vi "Copy Image Section.vi"(8 "Error In":errorcluster, 9 "Index to Copy (row, column)":cluster{"x":i16, "y":i16}, 10 "Pasteboard Picture":picture, 11 "Copy Picture":picture) -> (0 "Error Out":errorcluster, 3 "Output Picture":picture)   [LabVIEW 2011]
doc: "Copies a 50px by 50px box specified by a (row, column) index over a copy of the pasteboard picture onto a new picture."
panel:
  # "50px x 50px Subset"
  # "+"
  # "="
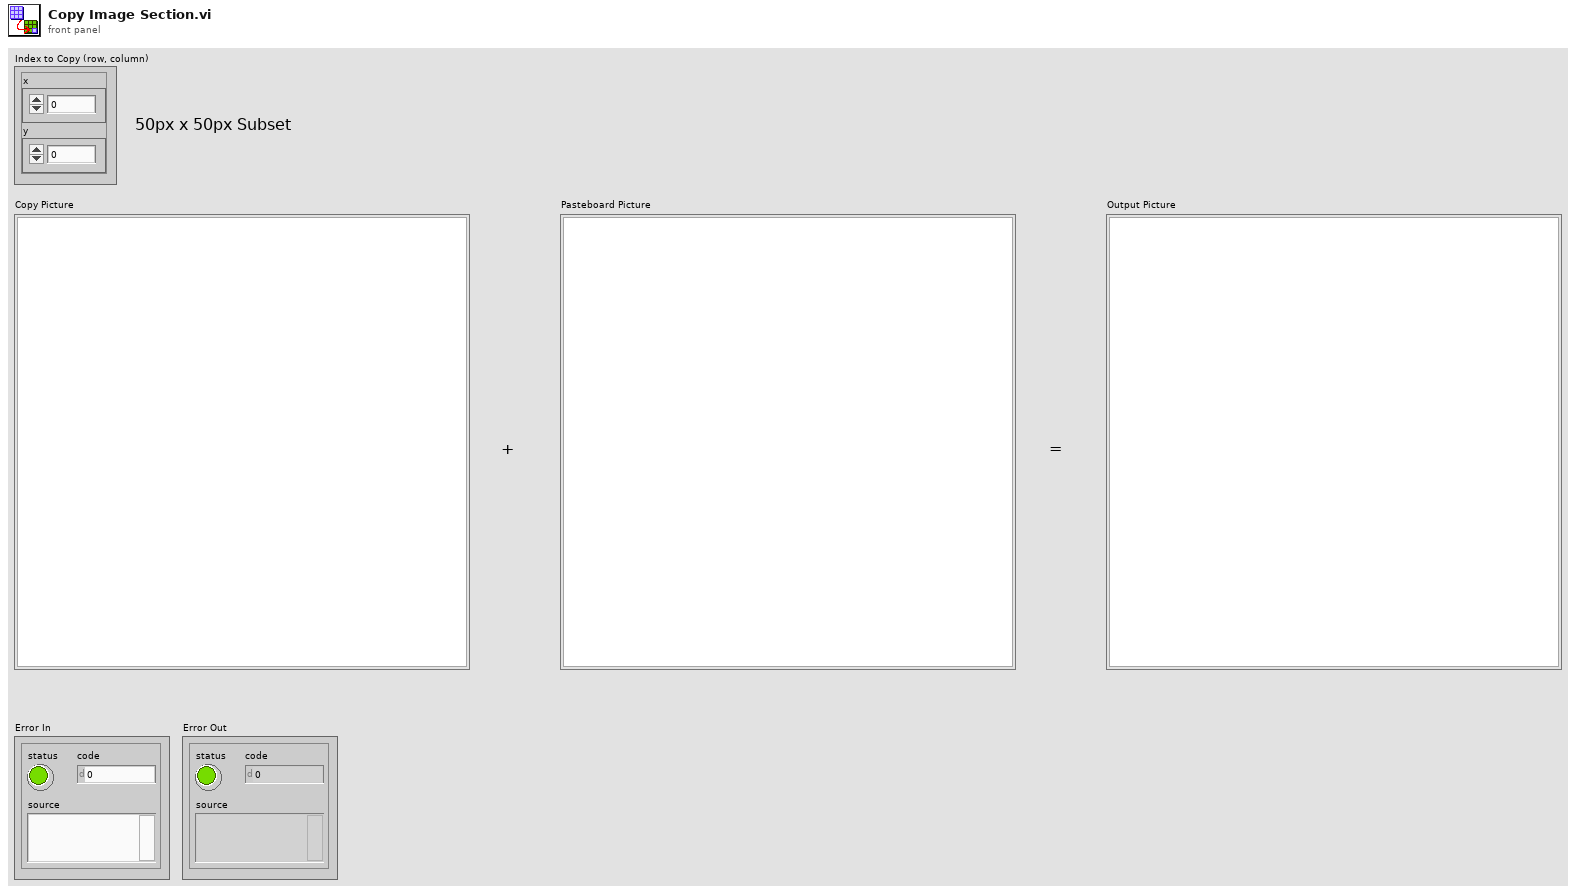
[diagram p1: front panel]
types:
  T1 = cluster{"left":i16, "top":i16, "right":i16, "bottom":i16}
  T2 = typedef "imagedata.ctl" = cluster{"image type":i32, "image depth":i32, "image":u8[], "mask":u8[], "colors":u32[], "Rectangle":cluster{"left":i16, "top":i16, "right":i16, "bottom":i16}}
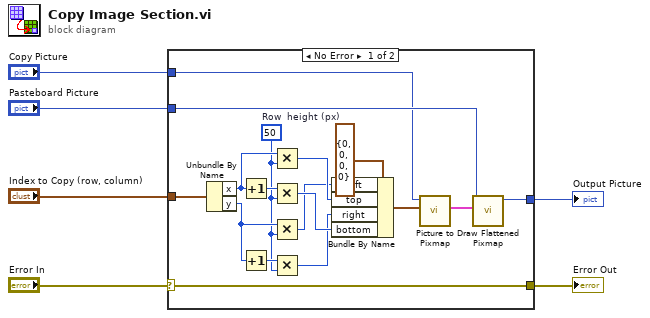
[diagram p0: block diagram]
diagram:
  n1 = case shown="No Error" "Error In" {
    selector: "Error In" -> [w7 w24]
    tunnel: "Index to Copy (row, column)" -> [w23 _]
    tunnel: "Pasteboard Picture" -> [w11 w25]
    tunnel: [w9 w25] -> w4
    tunnel: "Copy Picture" -> [w8 _]
    tunnel: [w7 w24] -> w1
    frame No Error {
      w18 = i16 50  # Row  height (px)
      n2 = Unbundle By Name(w23) -> ("x"=w22:i16, "y"=w20:i16)
      n3 = Increment(x=w22) -> (x+1=w21:i16)
      n4 = Increment(x=w20) -> (x+1=w19:i16)
      n5 = Multiply(x=w22, y=w18) -> (x*y=w17:i16)
      n6 = Multiply(x=w21, y=w18) -> (x*y=w16:i16)
      n7 = Multiply(x=w20, y=w18) -> (x*y=w15:i16)
      n8 = Multiply(x=w19, y=w18) -> (x*y=w14:i16)
      n9 = Bundle By Name(cluster=T1 {"left"=0, "top"=0, "right"=0, "bottom"=0} ("rect"), "left"=w15, "top"=w17, "right"=w14, "bottom"=w16) -> (w12:T1)
      n10 = call <vilib>:"Picture to Pixmap.vi"("rect"=w12, "picture"=w8) -> ("image data"=w10:T2)  [unwired: 8 in, 1 out]
      n11 = call <vilib>:"Draw Flattened Pixmap.vi"("image data"=w10, "picture"=w11) -> ("new picture"=w9:picture)  [unwired: 7 in]
    }
    frame Error {
    }
  }
  "Output Picture" <- w4
  "Error Out" <- w1
